vi "MW setup.vi"(11 "mw":T1={"mw_source"=enum."rigol", "MW Source IP Address"="169.254.101.2", "Remote Port"=18, "Frequency(MHz)"=1355.0, "Power(dBm)"=-27.0}) -> ()   [LabVIEW 2020]
uses:
  mw.ctl
  Labview Library/Libraries/HW_Rigol_DSG/Rigol Signal Generator Module/Rigol Signal Generator Module.lvlib
panel:
  out "error out":errorcluster
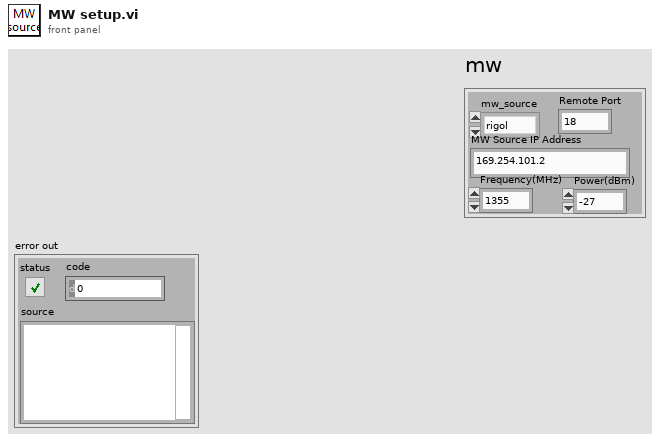
[diagram p1: front panel]
types:
  T1 = typedef "mw.ctl" = cluster{"mw_source":enum16{"rigol", "stanford", "apsin", "hittle"}, "MW Source IP Address":string, "Remote Port":u16, "Frequency(MHz)":dbl, "Power(dBm)":dbl}
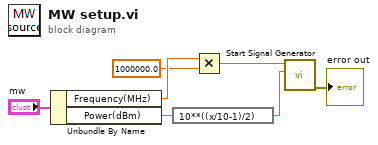
[diagram p0: block diagram]
diagram:
  n1 = Unbundle By Name("mw") -> ("Frequency(MHz)"=w3:dbl, "Power(dBm)"=w6:dbl)
  n2 = expression code="10**((x/10-1)/2)"(w6) -> (w5:dbl)
  n3 = Multiply(x=w3, y=1000000.0) -> (x*y=w1:dbl)
  n4 = call "Start Signal Generator.vi"("Amplitude (V)"=w5, "Frequency (Hz)"=w1) -> ("error out"=→"error out":errorcluster)  [unwired: 8 in, 1 out]
